vi "calc_AxisLengthMax.vi"(2 "# steps":u16=20 step=1 format="%#.0f", 3 "Step size":dbl=60.0 min=0.0, 4 "Minimum":dbl=33849.9 min=12000.0 max=62000.0 format="%#.2f") -> (0 "Maximum":dbl, 1 "Length":dbl)   [LabVIEW 2016]
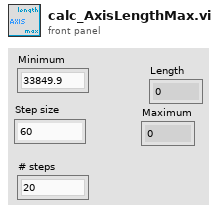
[diagram p1: front panel]
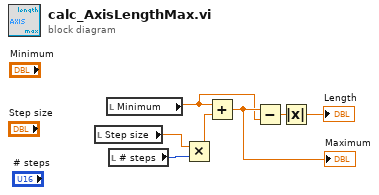
[diagram p0: block diagram]
diagram:
  n1 = local read "Step size"() -> (w7:dbl)
  n2 = local read "Minimum"() -> (w1:dbl)
  n3 = local read "# steps"() -> (w6:u16)
  n4 = Multiply(x=w7, y=w6) -> (x*y=w5:dbl)
  n5 = Add(x=w1, y=w5) -> (x+y=w2:dbl)
  "Maximum" <- w2
  n6 = Subtract(x=w2, y=w1) -> (x-y=w4:dbl)
  n7 = Absolute Value(x=w4) -> (abs(x)=→"Length":dbl)
